vi "async metadata user payload.vi"(8 "error in (no error)":errorcluster, 10 "user_payload_out":u32[](array[numeric])=[0, 0, 0, 0], 11 "h":u64) -> (0 "error out":errorcluster, 1 "function return":u32(ring), 2 "user_payload_out out":u32[](array[numeric]), 3 "h out":u64)   [LabVIEW 2023, in "uhd.lvlib"]
doc: "UHD_API uhd_error uhd_async_metadata_user_payload(\n uhd_async_metadata_handle h, uint32_t user_payload_out[4]);"
uses:
  <userlib>/uhd/uhd.lvlib
  <userlib>/uhd/uhd.dll
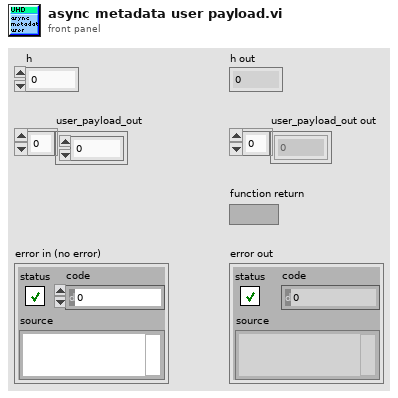
[diagram p1: front panel]
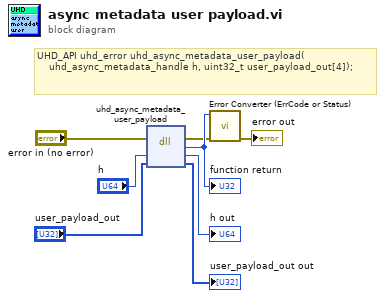
[diagram p0: block diagram]
diagram:
  # "UHD_API uhd_error uhd_async_metadata_user_payload(\n    uhd_async_metadata_handle h, uint32_t user_payload_out[4]);"
  n1 = dll-call lib="C:/Program Files/National Instruments/LabVIEW 2023/user.lib/uhd/uhd.*" fn="uhd_async_metadata_user_payload"(error in="error in (no error)", "h"="h", "user_payload_out"="user_payload_out") -> (error out=w2:errorcluster, w8:u32, "h"=→"h out":u64, "user_payload_out"=→"user_payload_out out":u32[])  [unwired: 2 in, 1 out]
  "function return" <- w8
  n2 = call <userlib>:"Error Converter (ErrCode or Status).vi"("error in (no error)"=w2, "error code"=w8) -> ("error out"=→"error out":errorcluster)  [unwired: 9 in]
